vi "LTE Fetch ACP.vi"(0 "RFmx Handle In":refnum<k21>, 1 "Selector String":string, 11 "error in (no error)":errorcluster) -> (4 "RFmx Handle Out":refnum<k21>, 6 "ACP Results":T1, 15 "error out":errorcluster)   [LabVIEW 2016, in "RFmxLTE.lvlib"]
uses:
  RFmxLTE.lvlib
  Typedefs/LTE ACP Results.ctl
  Typedefs/LTE ACP Offset Results.ctl
  Typedefs/LTE ACP Component Carrier Results.ctl
  <vilib>/RFmx/LTE/mx/RFmxLTE.llb/RFmxLTE ACP Fetch Offset Measurement (Array).vi
  <vilib>/RFmx/LTE/mx/RFmxLTE.llb/RFmxLTE ACP Fetch Component Carrier Measurement (Array).vi
  <resource>/objmgr/RFmxLTE.rc
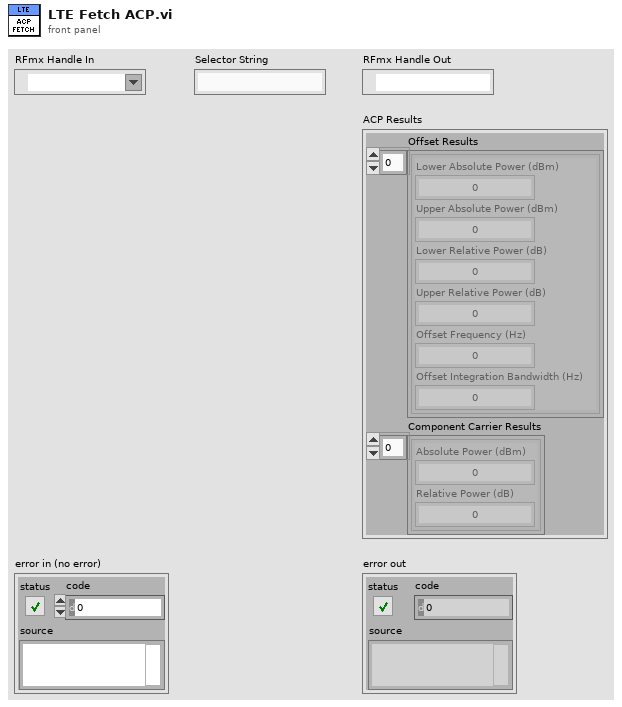
[diagram p1: front panel]
types:
  T1 = typedef "RFmxLTE.lvlib/LTE ACP Results.ctl" = cluster{"Offset Results":T2[], "Component Carrier Results":T3[]}
  T2 = typedef "RFmxLTE.lvlib/LTE ACP Offset Results.ctl" = cluster{"Lower Absolute Power (dBm)":dbl, "Upper Absolute Power (dBm)":dbl, "Lower Relative Power (dB)":dbl, "Upper Relative Power (dB)":dbl, "Offset Frequency (Hz)":dbl, "Offset Integration Bandwidth (Hz)":dbl}
  T3 = typedef "RFmxLTE.lvlib/LTE ACP Component Carrier Results.ctl" = cluster{"Absolute Power (dBm)":dbl, "Relative Power (dB)":dbl}
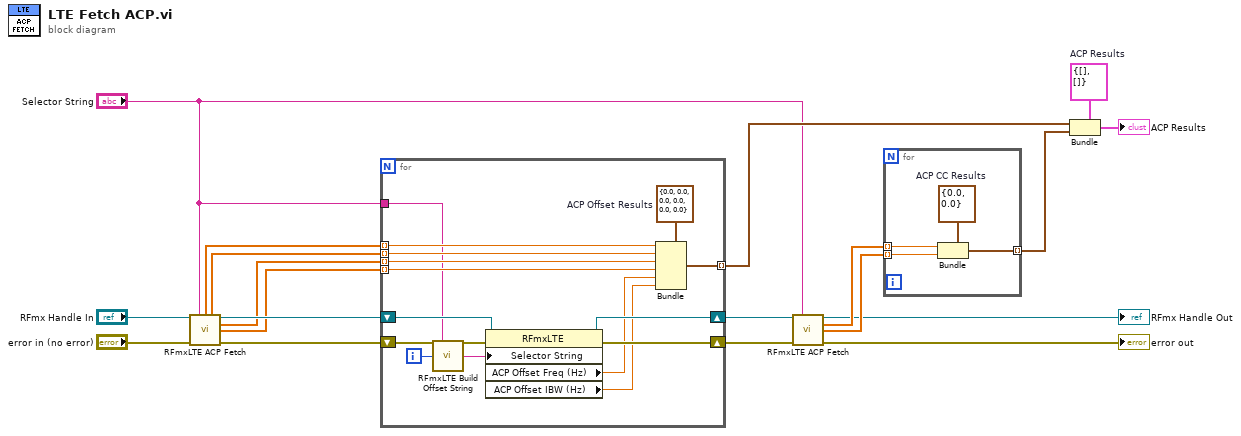
[diagram p0: block diagram]
diagram:
  w19 = T1 {"Offset Results"=[], "Component Carrier Results"=[]}  # ACP Results
  n1 = call-poly <vilib>:"RFmxLTE ACP Fetch.vi"("Instrument Handle In"="RFmx Handle In", "Selector String"="Selector String", "error in (no error)"="error in (no error)") -> ("Lower Absolute Power (dBm)"=w11:dbl[], "Upper Absolute Power (dBm)"=w10:dbl[], "Instrument Handle Out"=w13:refnum<k21>, "Lower Relative Power (dB)"=w9:dbl[], "Upper Relative Power (dB)"=w8:dbl[], "error out"=w12:errorcluster)  [unwired: 7 in]
  n2 = for {
    shift-right: [w32] -> w7
    shift-left: w13 -> [w26]
    shift-right: [w33] -> w6
    shift-left: w12 -> [w25]
    tunnel: [w28] -> w16 mode=indexing
    tunnel: w11 -> [w24] mode=indexing
    tunnel: w10 -> [w23] mode=indexing
    tunnel: w9 -> [w22] mode=indexing
    tunnel: w8 -> [w21] mode=indexing
    tunnel: "Selector String" -> [w20]
    i -> [w34]
    w31 = T2 {"Lower Absolute Power (dBm)"=0.0, "Upper Absolute Power (dBm)"=0.0, "Lower Relative Power (dB)"=0.0, "Upper Relative Power (dB)"=0.0, "Offset Frequency (Hz)"=0.0, "Offset Integration Bandwidth (Hz)"=0.0}  # ACP Offset Results
    n3 = call <vilib>:"RFmxLTE Build Offset String.vi"("Selector String"=w20, "Offset Number"=w34) -> ("Selector String Out"=w27:string)  [unwired: 13 in]
    n4 = property class="RFmxLTE"(reference=w26, error in=w25, "Selector String"=w27) -> (reference out=w32:refnum<k21>, error out=w33:errorcluster, "ACP Offset Freq (Hz)"=w29:dbl, "ACP Offset IBW (Hz)"=w30:dbl)
    n5 = Bundle(cluster=w31, "Lower Absolute Power (dBm)"=w24, "Upper Absolute Power (dBm)"=w23, "Lower Relative Power (dB)"=w22, "Upper Relative Power (dB)"=w21, "Offset Frequency (Hz)"=w29, "Offset Integration Bandwidth (Hz)"=w30) -> (w28:T2)
  }
  n6 = call-poly <vilib>:"RFmxLTE ACP Fetch.vi"("Instrument Handle In"=w7, "Selector String"="Selector String", "error in (no error)"=w6) -> ("Instrument Handle Out"=→"RFmx Handle Out":refnum<k21>, "Absolute Power (dBm)"=w5:dbl[], "Relative Power (dB)"=w4:dbl[], "error out"=→"error out":errorcluster)  [unwired: 9 in]
  n7 = for {
    tunnel: [w38] -> w17 mode=indexing
    tunnel: w5 -> [w36] mode=indexing
    tunnel: w4 -> [w35] mode=indexing
    w37 = T3 {"Absolute Power (dBm)"=0.0, "Relative Power (dB)"=0.0}  # ACP CC Results
    n8 = Bundle(cluster=w37, "Absolute Power (dBm)"=w36, "Relative Power (dB)"=w35) -> (w38:T3)
  }
  n9 = Bundle(cluster=w19, "Offset Results"=w16, "Component Carrier Results"=w17) -> (→"ACP Results":T1)
